vi "Aquisicao_NI_paralelo.vi"(4 "rate":dbl=3000.0 format="%0.2f", 5 "error in":errorcluster, 6 "Tempo de Aquisição":dbl, 7 "file path (dialog if empty)":path, 8 "task/channels in":refnum<k21>) -> (0 "error out":errorcluster, 1 "data":dbl[][](array[numeric]) format="%0.2f", 3 "task out":refnum<k21>)   [LabVIEW 2019]
uses:
  <vilib>/DAQmx/read.llb/DAQmx Read (Analog 2D DBL NChan NSamp).vi
  <vilib>/Utility/file.llb/Read Delimited Spreadsheet (string).vi
  <vilib>/Utility/file.llb/Write Delimited Spreadsheet (string).vi
  <vilib>/DAQmx/configure/timing.llb/DAQmx Timing (Sample Clock).vi
  <vilib>/DAQmx/miscellaneous.llb/DAQmx Fill In Error Info.vi
  <vilib>/Utility/file.llb/Write Delimited Spreadsheet (DBL).vi
panel:
  out "TimeStamp string":string
  out "Adquirindo":bool
  out "data size":i32[](array[numeric])
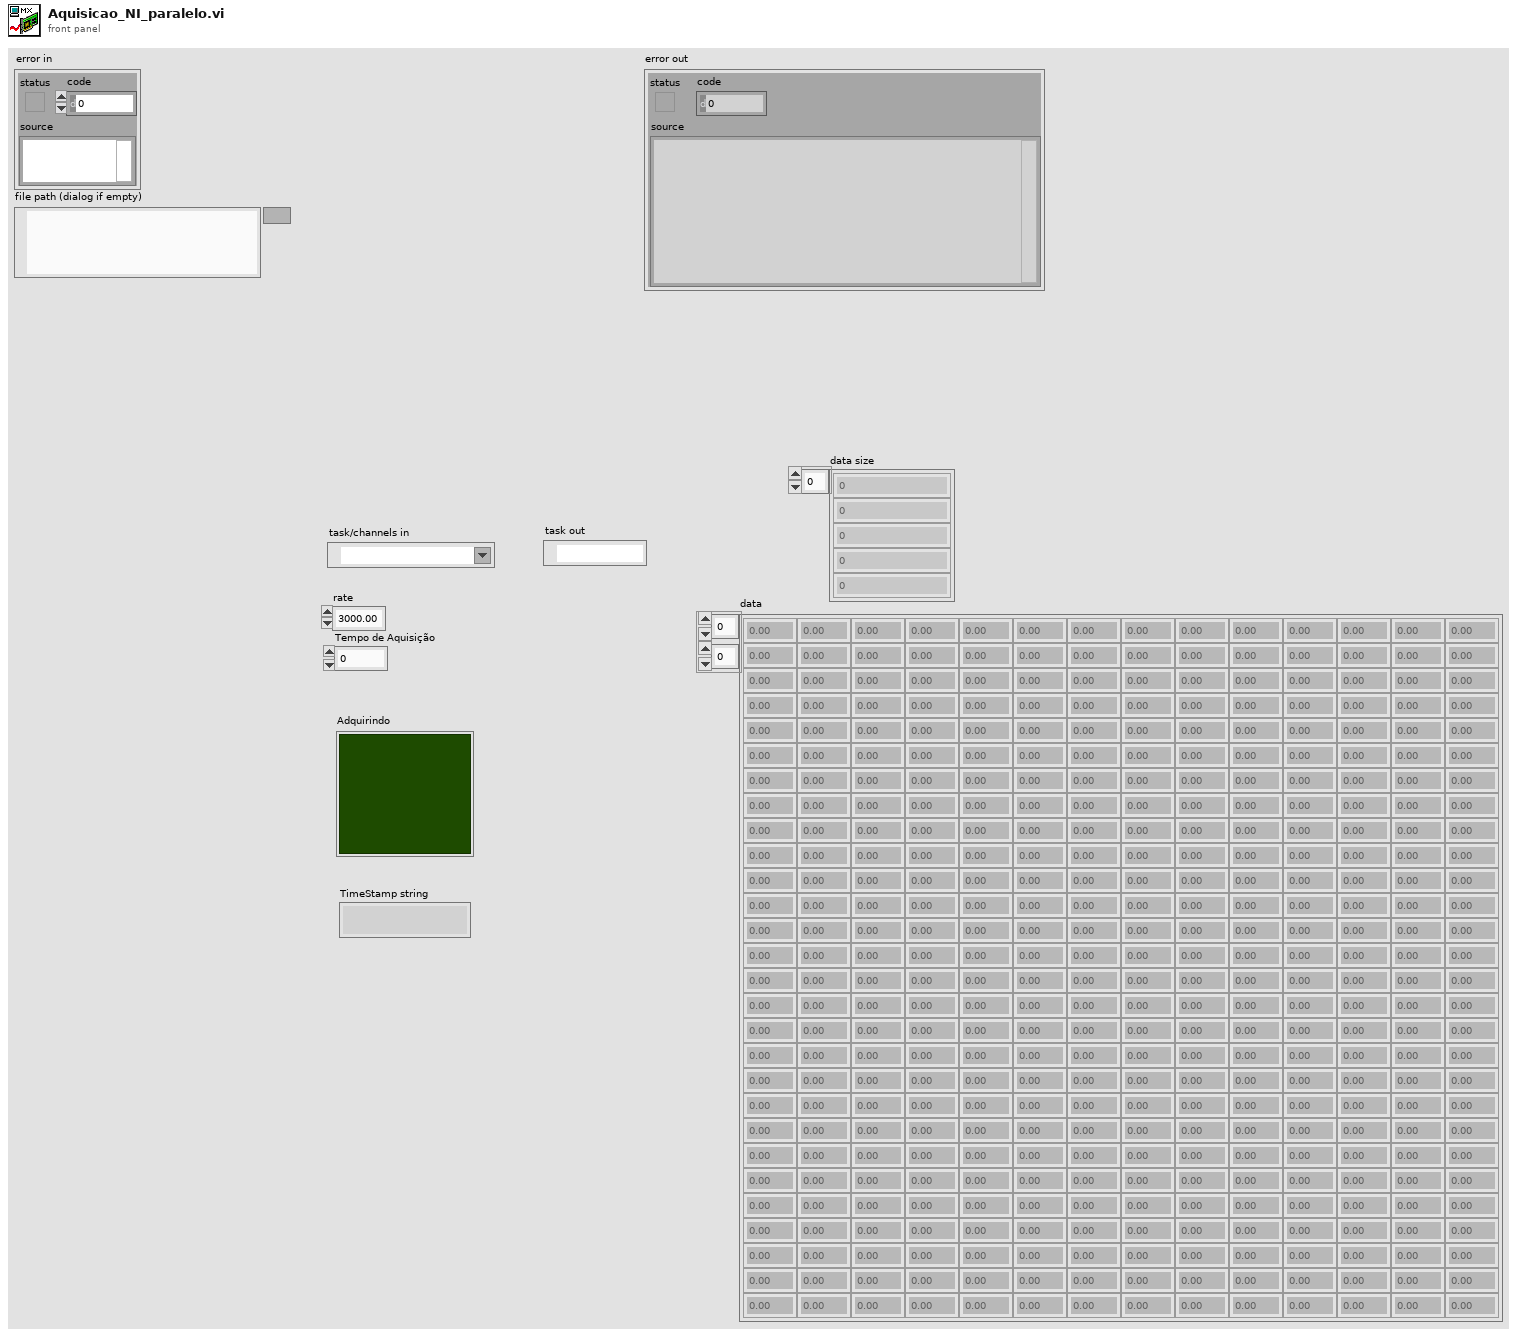
[diagram p1: front panel]
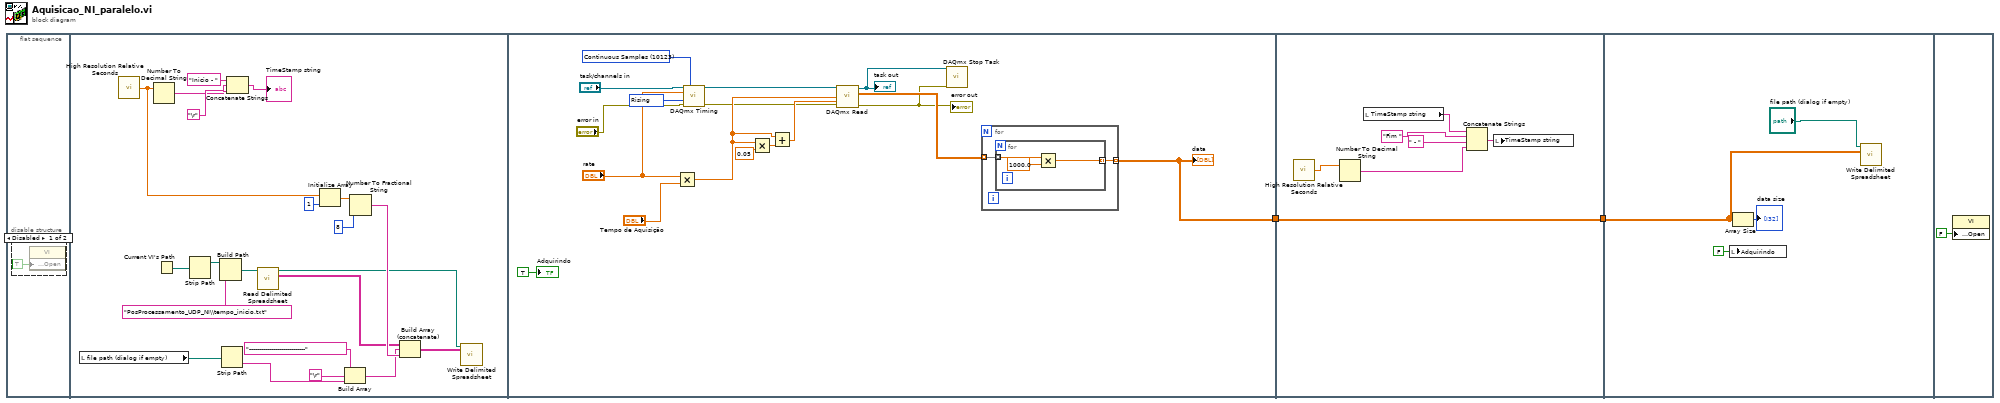
[diagram p0: block diagram]
diagram:
  n1 = flat-sequence {
    tunnel: [w29] -> w2
    tunnel: w2 -> [w53]
    tunnel: [w53] -> w1
    tunnel: w1 -> [w55]
    frame #0 {
      n2 = disable-structure shown="Disabled" {
        frame Disabled {
          n3 = property class="VI"("Front Panel.Open"=TRUE ("Front Panel Window:Open")) -> ()  [unwired: 2 in, 2 out]
        }
        frame Enabled {
        }
      }
    }
    frame #1 {
      n4 = local read "file path (dialog if empty)"() -> (w8:path)
      n5 = call <vilib>:"High Resolution Relative Seconds.vi"() -> ("relative seconds"=w10:dbl)
      n6 = Number To Decimal String(number=w10) -> (decimal integer string=w11:string)  [unwired: 1 in]
      n7 = Current VI's Path() -> (path=w13:path)
      n8 = Strip Path(path=w13) -> (stripped path=w12:path)  [unwired: 1 out]
      n9 = Build Path(base path=w12, name or relative path="PosProcessamento_UDP_NI\\tempo_inicio.txt") -> (appended path=w16:path)
      n10 = Strip Path(path=w8) -> (name=w7:string)  [unwired: 1 out]
      n11 = Concatenate Strings("Inicio - " ("string"), w11, "\r") -> (→"TimeStamp string":string)
      n12 = call-poly <vilib>:"Read Delimited Spreadsheet.vi"("file path (dialog if empty)"=w16) -> ("new file path (Not A Path if cancelled)"=w17:path, "all rows"=w9:string[][])  [unwired: 9 in, 4 out]
      n13 = Initialize Array(w10, 1 ("dimension size")) -> (w19:dbl[])
      n14 = Build Array("----------------------------" ("element"), "\r", w7) -> (w4:string[])
      n15 = Number To Fractional String(number=w19, precision (6)=i16 8) -> (F-format string=w20:string[])  [unwired: 2 in]
      n16 = Build Array (concatenate)(w9, w4, w20) -> (w15:string[][])
      n17 = call-poly <vilib>:"Write Delimited Spreadsheet.vi"("file path (dialog if empty)"=w17, "2D data"=w15) -> ()  [unwired: 12 in, 2 out]
    }
    frame #2 {
      w28 = 10280 items=["Rising"=10280, "Falling"=10171] ("active edge")
      w35 = 10123 items=["Finite Samples"=10178, "Continuous Samples"=10123, "Hardware Timed Single Point"=12522] ("sample mode")
      n18 = Multiply(x="rate", y="Tempo de Aquisição") -> (x*y=w38:dbl)
      n19 = call-poly <vilib>:"DAQmx Timing.vi"("task/channels in"="task/channels in", "sample mode"=w35, "rate"="rate", "active edge"=w28, "error in"="error in") -> ("task out"=w30:refnum<k21>, "error out"=w31:errorcluster)  [unwired: 9 in]
      n20 = Multiply(x=w38, y=0.05) -> (x*y=w40:dbl)
      n21 = Add(x=w38, y=w40) -> (x+y=w37:dbl)
      n22 = call-poly <vilib>:"DAQmx Read.vi"("task/channels in"=w30, "number of samples per channel"=w38, "timeout"=w37, "error in"=w31) -> ("task out"=w27:refnum<k21>, "data"=w36:dbl[][], "error out"=w26:errorcluster)  [unwired: 9 in]
      "task out" <- w27
      "error out" <- w26
      n23 = call <vilib>:"DAQmx Stop Task.vi"("task/channels in"=w27, "error in"=w26) -> ()  [unwired: 12 in, 2 out]
      n24 = for {
        tunnel: w36 -> [w43] mode=indexing
        tunnel: [w42] -> w29 mode=indexing
        n25 = for {
          tunnel: w43 -> [w46] mode=indexing
          tunnel: [w44] -> w42 mode=indexing
          n26 = Multiply(x=w46, y=1000.0) -> (x*y=w44:dbl)
        }
      }
      "data" <- w29
      "Adquirindo" <- TRUE ("Adquirindo")
    }
    frame #3 {
      n27 = call <vilib>:"High Resolution Relative Seconds.vi"() -> ("relative seconds"=w48:dbl)
      n28 = Number To Decimal String(number=w48) -> (decimal integer string=w47:string)  [unwired: 1 in]
      n29 = local read "TimeStamp string"() -> (w51:string)
      n30 = Concatenate Strings(w51, "Fim " ("string"), " - " ("string"), w47) -> (w52:string)
      n31 = local write "TimeStamp string"(w52) -> ()
    }
    frame #4 {
      n32 = local write "Adquirindo"(FALSE ("Adquirindo")) -> ()
      n33 = Array Size(array=w55) -> (size(s)=→"data size":i32[])
      n34 = call-poly <vilib>:"Write Delimited Spreadsheet.vi"("file path (dialog if empty)"="file path (dialog if empty)", "2D data"=w55) -> ()  [unwired: 12 in, 2 out]
    }
    frame #5 {
      n35 = property class="VI"("Front Panel.Open"=FALSE ("Front Panel Window:Open")) -> ()  [unwired: 2 in, 2 out]
    }
  }
